vi "PyTest.vi"() -> ()   [LabVIEW 2018]
panel:
  out "Cutelog PID":i32
  in  "Stop Cutelog":bool caption="Blandadk Button"
  in  "Start Cutelog":bool caption="Blandadk Button"
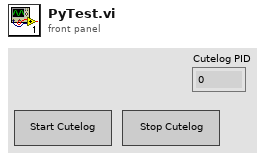
[diagram p1: front panel]
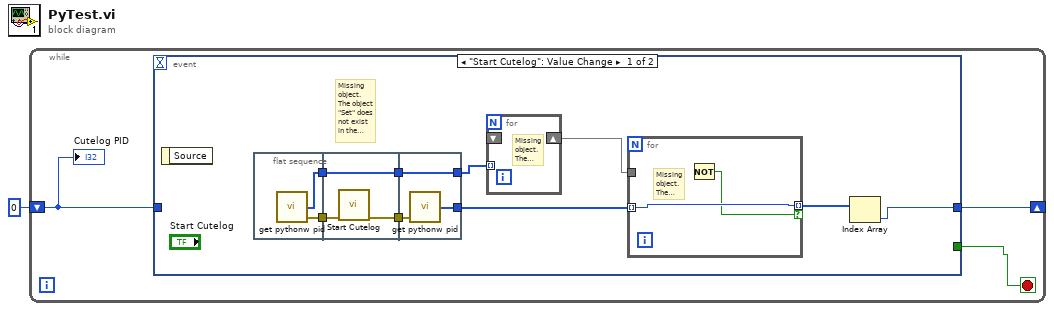
[diagram p0: block diagram]
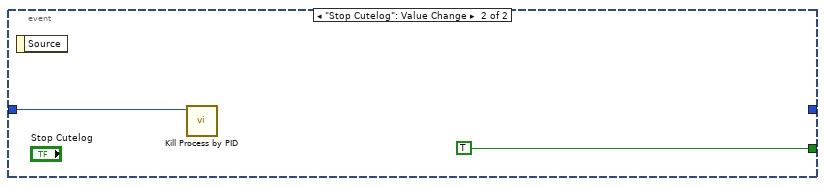
[diagram p2: hidden frame]
diagram:
  # "Missing object. The object \"Set\" does not exist in the previous version."
  n1 = while {
    shift-right: [w4] -> _
    shift-left: 0 -> [w3]
    stop <- w2 stop-if-true
    n2 = event shown="[0] \"Start Cutelog\": Value Change" {
      selector: _ -> [_ _]
      dyn-events: _ -> [_ _]
      timeout: _ -> [_ _]
      tunnel: [w8 _] -> w4
      tunnel: w3 -> [_ w26]
      tunnel: [_ TRUE] -> w2
      event "Start Cutelog": Value Change {
        n3 = event-data() -> ()  [unwired: 1 in, 1 out]
        n4 = flat-sequence {
          tunnel: [w18] -> w14
          tunnel: [w17] -> w13
          tunnel: w14 -> [w20]
          tunnel: [w21] -> w12
          tunnel: [w19] -> w11
          tunnel: w13 -> [w19]
          tunnel: w12 -> [w24]
          tunnel: [w23] -> w6
          tunnel: w11 -> [w23]
          tunnel: [w22] -> w10
          frame #0 {
            n5 = call "get pythonw pid.vi"() -> ("error out"=w18:errorcluster, "PIDs"=w17:i32[])  [unwired: 4 in]
          }
          frame #1 {
            n6 = call "Start Cutelog.vi"("error in (no error)"=w20) -> ("error out"=w21:errorcluster)  [unwired: 10 in]
          }
          frame #2 {
            n7 = call "get pythonw pid.vi"("error in (no error)"=w24) -> ("PIDs"=w22:i32[])  [unwired: 3 in, 1 out]
          }
        }
        n8 = for {
          tunnel: w6 -> [_] mode=indexing
          shift-right: [_] -> w5
          shift-left: [_] -> w7
          # "Missing object. The object \"Insert Into Set\" does not exist in the previous version."
        }
        n9 = for {
          tunnel: w10 -> [w16] mode=indexing
          tunnel: [w16] -> w9 mode=indexing if=w15
          tunnel: w5 -> [_]
          # "Missing object. The object \"Element of Set?\" does not exist in the previous version."
          n10 = Not() -> (.not. x?=w15:bool)  [unwired: 1 in]
        }
        n11 = Index Array(array=w9) -> (element=w8:i32)  [unwired: 1 in]
      }
      event "Stop Cutelog": Value Change {
        n12 = event-data() -> ()  [unwired: 1 in, 1 out]
        n13 = call "Kill Process by PID.vi"("PID"=w26) -> ()  [unwired: 10 in, 1 out]
      }
    }
    "Cutelog PID" <- w3
  }
